vi "FipsAdjacent.vi"() -> (11 "Fips":i32[](array[numeric]))   [LabVIEW 2017] (continued)
County, MN\"\t27105\n\"Lyon County, IA\"\t19119\t\"Rock County, MN\"\t27133\n\"Lyon County, IA\"\t19119\t\"Lincoln County, SD\"\t46083\n\"Lyon County, IA\"\t19119\t\"Minnehaha County, SD\"\t46099\n\"Madison County, IA\"\t19121\t\"Adair County, IA\"\t19001\n\"Madison County, IA\"\t19121\t\"Clarke County, IA\"\t19039\n\"Madison County, IA\"\t19121\t\"Dallas County, IA\"\t19049\n\"Madison County, IA\"\t19121\t\"Guthrie County, IA\"\t19077\n\"Madison County, IA\"\t19121\t\"Madison County, IA\"\t19121\n\"Madison County, IA\"\t19121\t\"Polk County, IA\"\t19153\n\"Madison County, IA\"\t19121\t\"Union County, IA\"\t19175\n\"Madison County, IA\"\t19121\t\"Warren County, IA\"\t19181\n\"Mahaska County, IA\"\t19123\t\"Jasper County, IA\"\t19099\n\"Mahaska County, IA\"\t19123\t\"Keokuk County, IA\"\t19107\n\"Mahaska County, IA\"\t19123\t\"Mahaska County, IA\"\t19123\n\"Mahaska County, IA\"\t19123\t\"Marion County, IA\"\t19125\n\"Mahaska County, IA\"\t19123\t\"Monroe County, IA\"\t19135\n\"Mahaska County, IA\"\t19123\t\"Poweshiek County, IA\"\t19157\n\"Mahaska County, IA\"\t19123\t\"Wapello County, IA\"\t19179\n\"Marion County, IA\"\t19125\t\"Jasper County, IA\"\t19099\n\"Marion County, IA\"\t19125\t\"Lucas County, IA\"\t19117\n\"Marion County, IA\"\t19125\t\"Mahaska County, IA\"\t19123\n\"Marion County, IA\"\t19125\t\"Marion County, IA\"\t19125\n\"Marion County, IA\"\t19125\t\"Monroe County, IA\"\t19135\n\"Marion County, IA\"\t19125\t\"Polk County, IA\"\t19153\n\"Marion County, IA\"\t19125\t\"Warren County, IA\"\t19181\n\"Marshall County, IA\"\t19127\t\"Grundy County, IA\"\t19075\n\"Marshall County, IA\"\t19127\t\"Hardin County, IA\"\t19083\n\"Marshall County, IA\"\t19127\t\"Jasper County, IA\"\t19099\n\"Marshall County, IA\"\t19127\t\"Marshall County, IA\"\t19127\n\"Marshall County, IA\"\t19127\t\"Poweshiek County, IA\"\t19157\n\"Marshall County, IA\"\t19127\t\"Story County, IA\"\t19169\n\"Marshall County, IA\"\t19127\t\"Tama County, IA\"\t19171\n\"Mills County, IA\"\t19129\t\"Fremont County, IA\"\t19071\n\"Mills County, IA\"\t19129\t\"Mills County, IA\"\t19129\n\"Mills County, IA\"\t19129\t\"Montgomery County, IA\"\t19137\n\"Mills County, IA\"\t19129\t\"Page County, IA\"\t19145\n\"Mills County, IA\"\t19129\t\"Pottawattamie County, IA\"\t19155\n\"Mills County, IA\"\t19129\t\"Cass County, NE\"\t31025\n\"Mills County, IA\"\t19129\t\"Sarpy County, NE\"\t31153\n\"Mitchell County, IA\"\t19131\t\"Cerro Gordo County, IA\"\t19033\n\"Mitchell County, IA\"\t19131\t\"Chickasaw County, IA\"\t19037\n\"Mitchell County, IA\"\t19131\t\"Floyd County, IA\"\t19067\n\"Mitchell County, IA\"\t19131\t\"Howard County, IA\"\t19089\n\"Mitchell County, IA\"\t19131\t\"Mitchell County, IA\"\t19131\n\"Mitchell County, IA\"\t19131\t\"Worth County, IA\"\t19195\n\"Mitchell County, IA\"\t19131\t\"Mower County, MN\"\t27099\n\"Monona County, IA\"\t19133\t\"Crawford County, IA\"\t19047\n\"Monona County, IA\"\t19133\t\"Harrison County, IA\"\t19085\n\"Monona County, IA\"\t19133\t\"Ida County, IA\"\t19093\n\"Monona County, IA\"\t19133\t\"Monona County, IA\"\t19133\n\"Monona County, IA\"\t19133\t\"Woodbury County, IA\"\t19193\n\"Monona County, IA\"\t19133\t\"Burt County, NE\"\t31021\n\"Monona County, IA\"\t19133\t\"Thurston County, NE\"\t31173\n\"Monroe County, IA\"\t19135\t\"Appanoose County, IA\"\t19007\n\"Monroe County, IA\"\t19135\t\"Davis County, IA\"\t19051\n\"Monroe County, IA\"\t19135\t\"Lucas County, IA\"\t19117\n\"Monroe County, IA\"\t19135\t\"Mahaska County, IA\"\t19123\n\"Monroe County, IA\"\t19135\t\"Marion County, IA\"\t19125\n\"Monroe County, IA\"\t19135\t\"Monroe County, IA\"\t19135\n\"Monroe County, IA\"\t19135\t\"Wapello County, IA\"\t19179\n\"Monroe County, IA\"\t19135\t\"Wayne County, IA\"\t19185\n\"Montgomery County, IA\"\t19137\t\"Adams County, IA\"\t19003\n\"Montgomery County, IA\"\t19137\t\"Cass County, IA\"\t19029\n\"Montgomery County, IA\"\t19137\t\"Fremont County, IA\"\t19071\n\"Montgomery County, IA\"\t19137\t\"Mills County, IA\"\t19129\n\"Montgomery County, IA\"\t19137\t\"Montgomery County, IA\"\t19137\n\"Montgomery County, IA\"\t19137\t\"Page County, IA\"\t19145\n\"Montgomery County, IA\"\t19137\t\"Pottawattamie County, IA\"\t19155\n\"Montgomery County, IA\"\t19137\t\"Taylor County, IA\"\t19173\n\"Muscatine County, IA\"\t19139\t\"Rock Island County, IL\"\t17161\n\"Muscatine County, IA\"\t19139\t\"Cedar County, IA\"\t19031\n\"Muscatine County, IA\"\t19139\t\"Johnson County, IA\"\t19103\n\"Muscatine County, IA\"\t19139\t\"Louisa County, IA\"\t19115\n\"Muscatine County, IA\"\t19139\t\"Muscatine County, IA\"\t19139\n\"Muscatine County, IA\"\t19139\t\"Scott County, IA\"\t19163\n\"O'Brien County, IA\"\t19141\t\"Buena Vista County, IA\"\t19021\n\"O'Brien County, IA\"\t19141\t\"Cherokee County, IA\"\t19035\n\"O'Brien County, IA\"\t19141\t\"Clay County, IA\"\t19041\n\"O'Brien County, IA\"\t19141\t\"Dickinson County, IA\"\t19059\n\"O'Brien County, IA\"\t19141\t\"Lyon County, IA\"\t19119\n\"O'Brien County, IA\"\t19141\t\"O'Brien County, IA\"\t19141\n\"O'Brien County, IA\"\t19141\t\"Osceola County, IA\"\t19143\n\"O'Brien County, IA\"\t19141\t\"Plymouth County, IA\"\t19149\n\"O'Brien County, IA\"\t19141\t\"Sioux County, IA\"\t19167\n\"Osceola County, IA\"\t19143\t\"Clay County, IA\"\t19041\n\"Osceola County, IA\"\t19143\t\"Dickinson County, IA\"\t19059\n\"Osceola County, IA\"\t19143\t\"Lyon County, IA\"\t19119\n\"Osceola County, IA\"\t19143\t\"O'Brien County, IA\"\t19141\n\"Osceola County, IA\"\t19143\t\"Osceola County, IA\"\t19143\n\"Osceola County, IA\"\t19143\t\"Sioux County, IA\"\t19167\n\"Osceola County, IA\"\t19143\t\"Jackson County, MN\"\t27063\n\"Osceola County, IA\"\t19143\t\"Nobles County, MN\"\t27105\n\"Page County, IA\"\t19145\t\"Adams County, IA\"\t19003\n\"Page County, IA\"\t19145\t\"Fremont County, IA\"\t19071\n\"Page County, IA\"\t19145\t\"Mills County, IA\"\t19129\n\"Page County, IA\"\t19145\t\"Montgomery County, IA\"\t19137\n\"Page County, IA\"\t19145\t\"Page County, IA\"\t19145\n\"Page County, IA\"\t19145\t\"Taylor County, IA\"\t19173\n\"Page County, IA\"\t19145\t\"Atchison County, MO\"\t29005\n\"Page County, IA\"\t19145\t\"Nodaway County, MO\"\t29147\n\"Palo Alto County, IA\"\t19147\t\"Buena Vista County, IA\"\t19021\n\"Palo Alto County, IA\"\t19147\t\"Clay County, IA\"\t19041\n\"Palo Alto County, IA\"\t19147\t\"Dickinson County, IA\"\t19059\n\"Palo Alto County, IA\"\t19147\t\"Emmet County, IA\"\t19063\n\"Palo Alto County, IA\"\t19147\t\"Humboldt County, IA\"\t19091\n\"Palo Alto County, IA\"\t19147\t\"Kossuth County, IA\"\t19109\n\"Palo Alto County, IA\"\t19147\t\"Palo Alto County, IA\"\t19147\n\"Palo Alto County, IA\"\t19147\t\"Pocahontas County, IA\"\t19151\n\"Plymouth County, IA\"\t19149\t\"Cherokee County, IA\"\t19035\n\"Plymouth County, IA\"\t19149\t\"O'Brien County, IA\"\t19141\n\"Plymouth County, IA\"\t19149\t\"Plymouth County, IA\"\t19149\n\"Plymouth County, IA\"\t19149\t\"Sioux County, IA\"\t19167\n\"Plymouth County, IA\"\t19149\t\"Woodbury County, IA\"\t19193\n\"Plymouth County, IA\"\t19149\t\"Union County, SD\"\t46127\n\"Pocahontas County, IA\"\t19151\t\"Buena Vista County, IA\"\t19021\n\"Pocahontas County, IA\"\t19151\t\"Calhoun County, IA\"\t19025\n\"Pocahontas County, IA\"\t19151\t\"Clay County, IA\"\t19041\n\"Pocahontas County, IA\"\t19151\t\"Humboldt County, IA\"\t19091\n\"Pocahontas County, IA\"\t19151\t\"Kossuth County, IA\"\t19109\n\"Pocahontas County, IA\"\t19151\t\"Palo Alto County, IA\"\t19147\n\"Pocahontas County, IA\"\t19151\t\"Pocahontas County, IA\"\t19151\n\"Pocahontas County, IA\"\t19151\t\"Sac County, IA\"\t19161\n\"Pocahontas County, IA\"\t19151\t\"Webster County, IA\"\t19187\n\"Polk County, IA\"\t19153\t\"Boone County, IA\"\t19015\n\"Polk County, IA\"\t19153\t\"Dallas County, IA\"\t19049\n\"Polk County, IA\"\t19153\t\"Jasper County, IA\"\t19099\n\"Polk County, IA\"\t19153\t\"Madison County, IA\"\t19121\n\"Polk County, IA\"\t19153\t\"Marion County, IA\"\t19125\n\"Polk County, IA\"\t19153\t\"Polk County, IA\"\t19153\n\"Polk County, IA\"\t19153\t\"Story County, IA\"\t19169\n\"Polk County, IA\"\t19153\t\"Warren County, IA\"\t19181\n\"Pottawattamie County, IA\"\t19155\t\"Cass County, IA\"\t19029\n\"Pottawattamie County, IA\"\t19155\t\"Harrison County, IA\"\t19085\n\"Pottawattamie County, IA\"\t19155\t\"Mills County, IA\"\t19129\n\"Pottawattamie County, IA\"\t19155\t\"Montgomery County, IA\"\t19137\n\"Pottawattamie County, IA\"\t19155\t\"Pottawattamie County, IA\"\t19155\n\"Pottawattamie County, IA\"\t19155\t\"Shelby County, IA\"\t19165\n\"Pottawattamie County, IA\"\t19155\t\"Douglas County, NE\"\t31055\n\"Pottawattamie County, IA\"\t19155\t\"Sarpy County, NE\"\t31153\n\"Pottawattamie County, IA\"\t19155\t\"Washington County, NE\"\t31177\n\"Poweshiek County, IA\"\t19157\t\"Benton County, IA\"\t19011\n\"Poweshiek County, IA\"\t19157\t\"Iowa County, IA\"\t19095\n\"Poweshiek County, IA\"\t19157\t\"Jasper County, IA\"\t19099\n\"Poweshiek County, IA\"\t19157\t\"Keokuk County, IA\"\t19107\n\"Poweshiek County, IA\"\t19157\t\"Mahaska County, IA\"\t19123\n\"Poweshiek County, IA\"\t19157\t\"Marshall County, IA\"\t19127\n\"Poweshiek County, IA\"\t19157\t\"Poweshiek County, IA\"\t19157\n\"Poweshiek County, IA\"\t19157\t\"Tama County, IA\"\t19171\n\"Ringgold County, IA\"\t19159\t\"Adams County, IA\"\t19003\n\"Ringgold County, IA\"\t19159\t\"Clarke County, IA\"\t19039\n\"Ringgold County, IA\"\t19159\t\"Decatur County, IA\"\t19053\n\"Ringgold County, IA\"\t19159\t\"Ringgold County, IA\"\t19159\n\"Ringgold County, IA\"\t19159\t\"Taylor County, IA\"\t19173\n\"Ringgold County, IA\"\t19159\t\"Union County, IA\"\t19175\n\"Ringgold County, IA\"\t19159\t\"Harrison County, MO\"\t29081\n\"Ringgold County, IA\"\t19159\t\"Worth County, MO\"\t29227\n\"Sac County, IA\"\t19161\t\"Buena Vista County, IA\"\t19021\n\"Sac County, IA\"\t19161\t\"Calhoun County, IA\"\t19025\n\"Sac County, IA\"\t19161\t\"Carroll County, IA\"\t19027\n\"Sac County, IA\"\t19161\t\"Cherokee County, IA\"\t19035\n\"Sac County, IA\"\t19161\t\"Crawford County, IA\"\t19047\n\"Sac County, IA\"\t19161\t\"Ida County, IA\"\t19093\n\"Sac County, IA\"\t19161\t\"Pocahontas County, IA\"\t19151\n\"Sac County, IA\"\t19161\t\"Sac County, IA\"\t19161\n\"Scott County, IA\"\t19163\t\"Rock Island County, IL\"\t17161\n\"Scott County, IA\"\t19163\t\"Cedar County, IA\"\t19031\n\"Scott County, IA\"\t19163\t\"Clinton County, IA\"\t19045\n\"Scott County, IA\"\t19163\t\"Muscatine County, IA\"\t19139\n\"Scott County, IA\"\t19163\t\"Scott County, IA\"\t19163\n\"Shelby County, IA\"\t19165\t\"Audubon County, IA\"\t19009\n\"Shelby County, IA\"\t19165\t\"Carroll County, IA\"\t19027\n\"Shelby County, IA\"\t19165\t\"Cass County, IA\"\t19029\n\"Shelby County, IA\"\t19165\t\"Crawford County, IA\"\t19047\n\"Shelby County, IA\"\t19165\t\"Harrison County, IA\"\t19085\n\"Shelby County, IA\"\t19165\t\"Pottawattamie County, IA\"\t19155\n\"Shelby County, IA\"\t19165\t\"Shelby County, IA\"\t19165\n\"Sioux County, IA\"\t19167\t\"Cherokee County, IA\"\t19035\n\"Sioux County, IA\"\t19167\t\"Lyon County, IA\"\t19119\n\"Sioux County, IA\"\t19167\t\"O'Brien County, IA\"\t19141\n\"Sioux County, IA\"\t19167\t\"Osceola County, IA\"\t19143\n\"Sioux County, IA\"\t19167\t\"Plymouth County, IA\"\t19149\n\"Sioux County, IA\"\t19167\t\"Sioux County, IA\"\t19167\n\"Sioux County, IA\"\t19167\t\"Lincoln County, SD\"\t46083\n\"Sioux County, IA\"\t19167\t\"Union County, SD\"\t46127\n\"Story County, IA\"\t19169\t\"Boone County, IA\"\t19015\n\"Story County, IA\"\t19169\t\"Hamilton County, IA\"\t19079\n\"Story County, IA\"\t19169\t\"Hardin County, IA\"\t19083\n\"Story County, IA\"\t19169\t\"Jasper County, IA\"\t19099\n\"Story County, IA\"\t19169\t\"Marshall County, IA\"\t19127\n\"Story County, IA\"\t19169\t\"Polk County, IA\"\t19153\n\"Story County, IA\"\t19169\t\"Story County, IA\"\t19169\n\"Tama County, IA\"\t19171\t\"Benton County, IA\"\t19011\n\"Tama County, IA\"\t19171\t\"Black Hawk County, IA\"\t19013\n\"Tama County, IA\"\t19171\t\"Grundy County, IA\"\t19075\n\"Tama County, IA\"\t19171\t\"Iowa County, IA\"\t19095\n\"Tama County, IA\"\t19171\t\"Jasper County, IA\"\t19099\n\"Tama County, IA\"\t19171\t\"Marshall County, IA\"\t19127\n\"Tama County, IA\"\t19171\t\"Poweshiek County, IA\"\t19157\n\"Tama County, IA\"\t19171\t\"Tama County, IA\"\t19171\n\"Taylor County, IA\"\t19173\t\"Adams County, IA\"\t19003\n\"Taylor County, IA\"\t19173\t\"Montgomery County, IA\"\t19137\n\"Taylor County, IA\"\t19173\t\"Page County, IA\"\t19145\n\"Taylor County, IA\"\t19173\t\"Ringgold County, IA\"\t19159\n\"Taylor County, IA\"\t19173\t\"Taylor County, IA\"\t19173\n\"Taylor County, IA\"\t19173\t\"Union County, IA\"\t19175\n\"Taylor County, IA\"\t19173\t\"Nodaway County, MO\"\t29147\n\"Taylor County, IA\"\t19173\t\"Worth County, MO\"\t29227\n\"Union County, IA\"\t19175\t\"Adair County, IA\"\t19001\n\"Union County, IA\"\t19175\t\"Adams County, IA\"\t19003\n\"Union County, IA\"\t19175\t\"Clarke County, IA\"\t19039\n\"Union County, IA\"\t19175\t\"Decatur County, IA\"\t19053\n\"Union County, IA\"\t19175\t\"Madison County, IA\"\t19121\n\"Union County, IA\"\t19175\t\"Ringgold County, IA\"\t19159\n\"Union County, IA\"\t19175\t\"Taylor County, IA\"\t19173\n\"Union County, IA\"\t19175\t\"Union County, IA\"\t19175\n\"Van Buren County, IA\"\t19177\t\"Davis County, IA\"\t19051\n\"Van Buren County, IA\"\t19177\t\"Henry County, IA\"\t19087\n\"Van Buren County, IA\"\t19177\t\"Jefferson County, IA\"\t19101\n\"Van Buren County, IA\"\t19177\t\"Lee County, IA\"\t19111\n\"Van Buren County, IA\"\t19177\t\"Van Buren County, IA\"\t19177\n\"Van Buren County, IA\"\t19177\t\"Wapello County, IA\"\t19179\n\"Van Buren County, IA\"\t19177\t\"Clark County, MO\"\t29045\n\"Van Buren County, IA\"\t19177\t\"Scotland County, MO\"\t29199\n\"Wapello County, IA\"\t19179\t\"Appanoose County, IA\"\t19007\n\"Wapello County, IA\"\t19179\t\"Davis County, IA\"\t19051\n\"Wapello County, IA\"\t19179\t\"Jefferson County, IA\"\t19101\n\"Wapello County, IA\"\t19179\t\"Keokuk County, IA\"\t19107\n\"Wapello County, IA\"\t19179\t\"Mahaska County, IA\"\t19123\n\"Wapello County, IA\"\t19179\t\"Monroe County, IA\"\t19135\n\"Wapello County, IA\"\t19179\t\"Van Buren County, IA\"\t19177\n\"Wapello County, IA\"\t19179\t\"Wapello County, IA\"\t19179\n\"Warren County, IA\"\t19181\t\"Clarke County, IA\"\t19039\n\"Warren County, IA\"\t19181\t\"Dallas County, IA\"\t19049\n\"Warren County, IA\"\t19181\t\"Lucas County, IA\"\t19117\n\"Warren County, IA\"\t19181\t\"Madison County, IA\"\t19121\n\"Warren County, IA\"\t19181\t\"Marion County, IA\"\t19125\n\"Warren County, IA\"\t19181\t\"Polk County, IA\"\t19153\n\"Warren County, IA\"\t19181\t\"Warren County, IA\"\t19181\n\"Washington County, IA\"\t19183\t\"Henry County, IA\"\t19087\n\"Washington County, IA\"\t19183\t\"Iowa County, IA\"\t19095\n\"Washington County, IA\"\t19183\t\"Jefferson County, IA\"\t19101\n\"Washington County, IA\"\t19183\t\"Johnson County, IA\"\t19103\n\"Washington County, IA\"\t19183\t\"Keokuk County, IA\"\t19107\n\"Washington County, IA\"\t19183\t\"Louisa County, IA\"\t19115\n\"Washington County, IA\"\t19183\t\"Washington County, IA\"\t19183\n\"Wayne County, IA\"\t19185\t\"Appanoose County, IA\"\t19007\n\"Wayne County, IA\"\t19185\t\"Clarke County, IA\"\t19039\n\"Wayne County, IA\"\t19185\t\"Decatur County, IA\"\t19053\n\"Wayne County, IA\"\t19185\t\"Lucas County, IA\"\t19117\n\"Wayne County, IA\"\t19185\t\"Monroe County, IA\"\t19135\n\"Wayne County, IA\"\t19185\t\"Wayne County, IA\"\t19185\n\"Wayne County, IA\"\t19185\t\"Mercer County, MO\"\t29129\n\"Wayne County, IA\"\t19185\t\"Putnam County, MO\"\t29171\n\"Webster County, IA\"\t19187\t\"Boone County, IA\"\t19015\n\"Webster County, IA\"\t19187\t\"Calhoun County, IA\"\t19025\n\"Webster County, IA\"\t19187\t\"Greene County, IA\"\t19073\n\"Webster County, IA\"\t19187\t\"Hamilton County, IA\"\t19079\n\"Webster County, IA\"\t19187\t\"Humboldt County, IA\"\t19091\n\"Webster County, IA\"\t19187\t\"Pocahontas County, IA\"\t19151\n\"Webster County, IA\"\t19187\t\"Webster County, IA\"\t19187\n\"Webster County, IA\"\t19187\t\"Wright County, IA\"\t19197\n\"Winnebago County, IA\"\t19189\t\"Cerro Gordo County, IA\"\t19033\n\"Winnebago County, IA\"\t19189\t\"Hancock County, IA\"\t19081\n\"Winnebago County, IA\"\t19189\t\"Kossuth County, IA\"\t19109\n\"Winnebago County, IA\"\t19189\t\"Winnebago County, IA\"\t19189\n\"Winnebago County, IA\"\t19189\t\"Worth County, IA\"\t19195\n\"Winnebago County, IA\"\t19189\t\"Faribault County, MN\"\t27043\n\"Winnebago County, IA\"\t19189\t\"Freeborn County, MN\"\t27047\n\"Winneshiek County, IA\"\t19191\t\"Allamakee County, IA\"\t19005\n\"Winneshiek County, IA\"\t19191\t\"Chickasaw County, IA\"\t19037\n\"Winneshiek County, IA\"\t19191\t\"Clayton County, IA\"\t19043\n\"Winneshiek County, IA\"\t19191\t\"Fayette County, IA\"\t19065\n\"Winneshiek County, IA\"\t19191\t\"Howard County, IA\"\t19089\n\"Winneshiek County, IA\"\t19191\t\"Winneshiek County, IA\"\t19191\n\"Winneshiek County, IA\"\t19191\t\"Fillmore County, MN\"\t27045\n\"Winneshiek County, IA\"\t19191\t\"Houston County, MN\"\t27055\n\"Woodbury County, IA\"\t19193\t\"Cherokee County, IA\"\t19035\n\"Woodbury County, IA\"\t19193\t\"Crawford County, IA\"\t19047\n\"Woodbury County, IA\"\t19193\t\"Ida County, IA\"\t19093\n\"Woodbury County, IA\"\t19193\t\"Monona County, IA\"\t19133\n\"Woodbury County, IA\"\t19193\t\"Plymouth County, IA\"\t19149\n\"Woodbury County, IA\"\t19193\t\"Woodbury County, IA\"\t19193\n\"Woodbury County, IA\"\t19193\t\"Dakota County, NE\"\t31043\n\"Woodbury County, IA\"\t19193\t\"Thurston County, NE\"\t31173\n\"Woodbury County, IA\"\t19193\t\"Union County, SD\"\t46127\n\"Worth County, IA\"\t19195\t\"Cerro Gordo County, IA\"\t19033\n\"Worth County, IA\"\t19195\t\"Hancock County, IA\"\t19081\n\"Worth County, IA\"\t19195\t\"Mitchell County, IA\"\t19131\n\"Worth County, IA\"\t19195\t\"Winnebago County, IA\"\t19189\n\"Worth County, IA\"\t19195\t\"Worth County, IA\"\t19195\n\"Worth County, IA\"\t19195\t\"Freeborn County, MN\"\t27047\n\"Worth County, IA\"\t19195\t\"Mower County, MN\"\t27099\n\"Wright County, IA\"\t19197\t\"Cerro Gordo County, IA\"\t19033\n\"Wright County, IA\"\t19197\t\"Franklin County, IA\"\t19069\n\"Wright County, IA\"\t19197\t\"Hamilton County, IA\"\t19079\n\"Wright County, IA\"\t19197\t\"Hancock County, IA\"\t19081\n\"Wright County, IA\"\t19197\t\"Hardin County, IA\"\t19083\n\"Wright County, IA\"\t19197\t\"Humboldt County, IA\"\t19091\n\"Wright County, IA\"\t19197\t\"Kossuth County, IA\"\t19109\n\"Wright County, IA\"\t19197\t\"Webster County, IA\"\t19187\n\"Wright County, IA\"\t19197\t\"Wright County, IA\"\t19197\n\"Allen County, KS\"\t20001\t\"Allen County, KS\"\t20001\n\"Allen County, KS\"\t20001\t\"Anderson County, KS\"\t20003\n\"Allen County, KS\"\t20001\t\"Bourbon County, KS\"\t20011\n\"Allen County, KS\"\t20001\t\"Coffey County, KS\"\t20031\n\"Allen County, KS\"\t20001\t\"Linn County, KS\"\t20107\n\"Allen County, KS\"\t20001\t\"Neosho County, KS\"\t20133\n\"Allen County, KS\"\t20001\t\"Wilson County, KS\"\t20205\n\"Allen County, KS\"\t20001\t\"Woodson County, KS\"\t20207\n\"Anderson County, KS\"\t20003\t\"Allen County, KS\"\t20001\n\"Anderson County, KS\"\t20003\t\"Anderson County, KS\"\t20003\n\"Anderson County, KS\"\t20003\t\"Bourbon County, KS\"\t20011\n\"Anderson County, KS\"\t20003\t\"Coffey County, KS\"\t20031\n\"Anderson County, KS\"\t20003\t\"Franklin County, KS\"\t20059\n\"Anderson County, KS\"\t20003\t\"Linn County, KS\"\t20107\n\"Anderson County, KS\"\t20003\t\"Miami County, KS\"\t20121\n\"Anderson County, KS\"\t20003\t\"Woodson County, KS\"\t20207\n\"Atchison County, KS\"\t20005\t\"Atchison County, KS\"\t20005\n\"Atchison County, KS\"\t20005\t\"Brown County, KS\"\t20013\n\"Atchison County, KS\"\t20005\t\"Doniphan County, KS\"\t20043\n\"Atchison County, KS\"\t20005\t\"Jackson County, KS\"\t20085\n\"Atchison County, KS\"\t20005\t\"Jefferson County, KS\"\t20087\n\"Atchison County, KS\"\t20005\t\"Leavenworth County, KS\"\t20103\n\"Atchison County, KS\"\t20005\t\"Buchanan County, MO\"\t29021\n\"Atchison County, KS\"\t20005\t\"Platte County, MO\"\t29165\n\"Barber County, KS\"\t20007\t\"Barber County, KS\"\t20007\n\"Barber County, KS\"\t20007\t\"Comanche County, KS\"\t20033\n\"Barber County, KS\"\t20007\t\"Harper County, KS\"\t20077\n\"Barber County, KS\"\t20007\t\"Kingman County, KS\"\t20095\n\"Barber County, KS\"\t20007\t\"Kiowa County, KS\"\t20097\n\"Barber County, KS\"\t20007\t\"Pratt County, KS\"\t20151\n\"Barber County, KS\"\t20007\t\"Alfalfa County, OK\"\t40003\n\"Barber County, KS\"\t20007\t\"Woods County, OK\"\t40151\n\"Barton County, KS\"\t20009\t\"Barton County, KS\"\t20009\n\"Barton County, KS\"\t20009\t\"Ellsworth County, KS\"\t20053\n\"Barton County, KS\"\t20009\t\"Pawnee County, KS\"\t20145\n\"Barton County, KS\"\t20009\t\"Rice County, KS\"\t20159\n\"Barton County, KS\"\t20009\t\"Rush County, KS\"\t20165\n\"Barton County, KS\"\t20009\t\"Russell County, KS\"\t20167\n\"Barton County, KS\"\t20009\t\"Stafford County, KS\"\t20185\n\"Bourbon County, KS\"\t20011\t\"Allen County, KS\"\t20001\n\"Bourbon County, KS\"\t20011\t\"Anderson County, KS\"\t20003\n\"Bourbon County, KS\"\t20011\t\"Bourbon County, KS\"\t20011\n\"Bourbon County, KS\"\t20011\t\"Crawford County, KS\"\t20037\n\"Bourbon County, KS\"\t20011\t\"Linn County, KS\"\t20107\n\"Bourbon County, KS\"\t20011\t\"Neosho County, KS\"\t20133\n\"Bourbon County, KS\"\t20011\t\"Vernon County, MO\"\t29217\n\"Brown County, KS\"\t20013\t\"Atchison County, KS\"\t20005\n\"Brown County, KS\"\t20013\t\"Brown County, KS\"\t20013\n\"Brown County, KS\"\t20013\t\"Doniphan County, KS\"\t20043\n\"Brown County, KS\"\t20013\t\"Jackson County, KS\"\t20085\n\"Brown County, KS\"\t20013\t\"Nemaha County, KS\"\t20131\n\"Brown County, KS\"\t20013\t\"Richardson County, NE\"\t31147\n\"Butler County, KS\"\t20015\t\"Butler County, KS\"\t20015\n\"Butler County, KS\"\t20015\t\"Chase County, KS\"\t20017\n\"Butler County, KS\"\t20015\t\"Cowley County, KS\"\t20035\n\"Butler County, KS\"\t20015\t\"Elk County, KS\"\t20049\n\"Butler County, KS\"\t20015\t\"Greenwood County, KS\"\t20073\n\"Butler County, KS\"\t20015\t\"Harvey County, KS\"\t20079\n\"Butler County, KS\"\t20015\t\"Marion County, KS\"\t20115\n\"Butler County, KS\"\t20015\t\"Sedgwick County, KS\"\t20173\n\"Butler County, KS\"\t20015\t\"Sumner County, KS\"\t20191\n\"Chase County, KS\"\t20017\t\"Butler County, KS\"\t20015\n\"Chase County, KS\"\t20017\t\"Chase County, KS\"\t20017\n\"Chase County, KS\"\t20017\t\"Greenwood County, KS\"\t20073\n\"Chase County, KS\"\t20017\t\"Lyon County, KS\"\t20111\n\"Chase County, KS\"\t20017\t\"Marion County, KS\"\t20115\n\"Chase County, KS\"\t20017\t\"Morris County, KS\"\t20127\n\"Chautauqua County, KS\"\t20019\t\"Chautauqua County, KS\"\t20019\n\"Chautauqua County, KS\"\t20019\t\"Cowley County, KS\"\t20035\n\"Chautauqua County, KS\"\t20019\t\"Elk County, KS\"\t20049\n\"Chautauqua County, KS\"\t20019\t\"Montgomery County, KS\"\t20125\n\"Chautauqua County, KS\"\t20019\t\"Osage County, OK\"\t40113\n\"Chautauqua County, KS\"\t20019\t\"Washington County, OK\"\t40147\n\"Cherokee County, KS\"\t20021\t\"Cherokee County, KS\"\t20021\n\"Cherokee County, KS\"\t20021\t\"Crawford County, KS\"\t20037\n\"Cherokee County, KS\"\t20021\t\"Labette County, KS\"\t20099\n\"Cherokee County, KS\"\t20021\t\"Jasper County, MO\"\t29097\n\"Cherokee County, KS\"\t20021\t\"Newton County, MO\"\t29145\n\"Cherokee County, KS\"\t20021\t\"Craig County, OK\"\t40035\n\"Cherokee County, KS\"\t20021\t\"Ottawa County, OK\"\t40115\n\"Cheyenne County, KS\"\t20023\t\"Kit Carson County, CO\"\t08063\n\"Cheyenne County, KS\"\t20023\t\"Yuma County, CO\"\t08125\n\"Cheyenne County, KS\"\t20023\t\"Cheyenne County, KS\"\t20023\n\"Cheyenne County, KS\"\t20023\t\"Rawlins County, KS\"\t20153\n\"Cheyenne County, KS\"\t20023\t\"Sherman County, KS\"\t20181\n\"Cheyenne County, KS\"\t20023\t\"Dundy County, NE\"\t31057\n\"Clark County, KS\"\t20025\t\"Clark County, KS\"\t20025\n\"Clark County, KS\"\t20025\t\"Comanche County, KS\"\t20033\n\"Clark County, KS\"\t20025\t\"Ford County, KS\"\t20057\n\"Clark County, KS\"\t20025\t\"Kiowa County, KS\"\t20097\n\"Clark County, KS\"\t20025\t\"Meade County, KS\"\t20119\n\"Clark County, KS\"\t20025\t\"Beaver County, OK\"\t40007\n\"Clark County, KS\"\t20025\t\"Harper County, OK\"\t40059\n\"Clay County, KS\"\t20027\t\"Clay County, KS\"\t20027\n\"Clay County, KS\"\t20027\t\"Cloud County, KS\"\t20029\n\"Clay County, KS\"\t20027\t\"Dickinson County, KS\"\t20041\n\"Clay County, KS\"\t20027\t\"Geary County, KS\"\t20061\n\"Clay County, KS\"\t20027\t\"Ottawa County, KS\"\t20143\n\"Clay County, KS\"\t20027\t\"Riley County, KS\"\t20161\n\"Clay County, KS\"\t20027\t\"Washington County, KS\"\t20201\n\"Cloud County, KS\"\t20029\t\"Clay County, KS\"\t20027\n\"Cloud County, KS\"\t20029\t\"Cloud County, KS\"\t20029\n\"Cloud County, KS\"\t20029\t\"Jewell County, KS\"\t20089\n\"Cloud County, KS\"\t20029\t\"Mitchell County, KS\"\t20123\n\"Cloud County, KS\"\t20029\t\"Ottawa County, KS\"\t20143\n\"Cloud County, KS\"\t20029\t\"Republic County, KS\"\t20157\n\"Cloud County, KS\"\t20029\t\"Washington County, KS\"\t20201\n\"Coffey County, KS\"\t20031\t\"Allen County, KS\"\t20001\n\"Coffey County, KS\"\t20031\t\"Anderson County, KS\"\t20003\n\"Coffey County, KS\"\t20031\t\"Coffey County, KS\"\t20031\n\"Coffey County, KS\"\t20031\t\"Franklin County, KS\"\t20059\n\"Coffey County, KS\"\t20031\t\"Greenwood County, KS\"\t20073\n\"Coffey County, KS\"\t20031\t\"Lyon County, KS\"\t20111\n\"Coffey County, KS\"\t20031\t\"Osage County, KS\"\t20139\n\"Coffey County, KS\"\t20031\t\"Woodson County, KS\"\t20207\n\"Comanche County, KS\"\t20033\t\"Barber County, KS\"\t20007\n\"Comanche County, KS\"\t20033\t\"Clark County, KS\"\t20025\n\"Comanche County, KS\"\t20033\t\"Comanche County, KS\"\t20033\n\"Comanche County, KS\"\t20033\t\"Kiowa County, KS\"\t20097\n\"Comanche County, KS\"\t20033\t\"Harper County, OK\"\t40059\n\"Comanche County, KS\"\t20033\t\"Woods County, OK\"\t40151\n\"Cowley County, KS\"\t20035\t\"Butler County, KS\"\t20015\n\"Cowley County, KS\"\t20035\t\"Chautauqua County, KS\"\t20019\n\"Cowley County, KS\"\t20035\t\"Cowley County, KS\"\t20035\n\"Cowley County, KS\"\t20035\t\"Elk County, KS\"\t20049\n\"Cowley County, KS\"\t20035\t\"Sedgwick County, KS\"\t20173\n\"Cowley County, KS\"\t20035\t\"Sumner County, KS\"\t20191\n\"Cowley County, KS\"\t20035\t\"Kay County, OK\"\t40071\n\"Cowley County, KS\"\t20035\t\"Osage County, OK\"\t40113\n\"Crawford County, KS\"\t20037\t\"Bourbon County, KS\"\t20011\n\"Crawford County, KS\"\t20037\t\"Cherokee County, KS\"\t20021\n\"Crawford County, KS\"\t20037\t\"Crawford County, KS\"\t20037\n\"Crawford County, KS\"\t20037\t\"Labette County, KS\"\t20099\n\"Crawford County, KS\"\t20037\t\"Neosho County, KS\"\t20133\n\"Crawford County, KS\"\t20037\t\"Barton County, MO\"\t29011\n\"Crawford County, KS\"\t20037\t\"Jasper County, MO\"\t29097\n\"Crawford County, KS\"\t20037\t\"Vernon County, MO\"\t29217\n\"Decatur County, KS\"\t20039\t\"Decatur County, KS\"\t20039\n\"Decatur County, KS\"\t20039\t\"Norton County, KS\"\t20137\n\"Decatur County, KS\"\t20039\t\"Rawlins County, KS\"\t20153\n\"Decatur County, KS\"\t20039\t\"Sheridan County, KS\"\t20179\n\"Decatur County, KS\"\t20039\t\"Thomas County, KS\"\t20193\n\"Decatur County, KS\"\t20039\t\"Furnas County, NE\"\t31065\n\"Decatur County, KS\"\t20039\t\"Red Willow County, NE\"\t31145\n\"Dickinson County, KS\"\t20041\t\"Clay County, KS\"\t20027\n\"Dickinson County, KS\"\t20041\t\"Dickinson County, KS\"\t20041\n\"Dickinson County, KS\"\t20041\t\"Geary County, KS\"\t20061\n\"Dickinson County, KS\"\t20041\t\"McPherson County, KS\"\t20113\n\"Dickinson County, KS\"\t20041\t\"Marion County, KS\"\t20115\n\"Dickinson County, KS\"\t20041\t\"Morris County, KS\"\t20127\n\"Dickinson County, KS\"\t20041\t\"Ottawa County, KS\"\t20143\n\"Dickinson County, KS\"\t20041\t\"Saline County, KS\"\t20169\n\"Doniphan County, KS\"\t20043\t\"Atchison County, KS\"\t20005\n\"Doniphan County, KS\"\t20043\t\"Brown County, KS\"\t20013\n\"Doniphan County, KS\"\t20043\t\"Doniphan County, KS\"\t20043\n\"Doniphan County, KS\"\t20043\t\"Andrew County, MO\"\t29003\n\"Doniphan County, KS\"\t20043\t\"Buchanan County, MO\"\t29021\n\"Doniphan County, KS\"\t20043\t\"Holt County, MO\"\t29087\n\"Doniphan County, KS\"\t20043\t\"Richardson County, NE\"\t31147\n\"Douglas County, KS\"\t20045\t\"Douglas County, KS\"\t20045\n\"Douglas County, KS\"\t20045\t\"Franklin County, KS\"\t20059\n\"Douglas County, KS\"\t20045\t\"Jefferson County, KS\"\t20087\n\"Douglas County, KS\"\t20045\t\"Johnson County, KS\"\t20091\n\"Douglas County, KS\"\t20045\t\"Leavenworth County, KS\"\t20103\n\"Douglas County, KS\"\t20045\t\"Miami County, KS\"\t20121\n\"Douglas County, KS\"\t20045\t\"Osage County, KS\"\t20139\n\"Douglas County, KS\"\t20045\t\"Shawnee County, KS\"\t20177\n\"Edwards County, KS\"\t20047\t\"Edwards County, KS\"\t20047\n\"Edwards County, KS\"\t20047\t\"Ford County, KS\"\t20057\n\"Edwards County, KS\"\t20047\t\"Hodgeman County, KS\"\t20083\n\"Edwards County, KS\"\t20047\t\"Kiowa County, KS\"\t20097\n\"Edwards County, KS\"\t20047\t\"Pawnee County, KS\"\t20145\n\"Edwards County, KS\"\t20047\t\"Pratt County, KS\"\t20151\n\"Edwards County, KS\"\t20047\t\"Stafford County, KS\"\t20185\n\"Elk County, KS\"\t20049\t\"Butler County, KS\"\t20015\n\"Elk County, KS\"\t20049\t\"Chautauqua County, KS\"\t20019\n\"Elk County, KS\"\t20049\t\"Cowley County, KS\"\t20035\n\"Elk County, KS\"\t20049\t\"Elk County, KS\"\t20049\n\"Elk County, KS\"\t20049\t\"Greenwood County, KS\"\t20073\n\"Elk County, KS\"\t20049\t\"Montgomery County, KS\"\t20125\n\"Elk County, KS\"\t20049\t\"Wilson County, KS\"\t20205\n\"Ellis County, KS\"\t20051\t\"Ellis County, KS\"\t20051\n\"Ellis County, KS\"\t20051\t\"Ness County, KS\"\t20135\n\"Ellis County, KS\"\t20051\t\"Osborne County, KS\"\t20141\n\"Ellis County, KS\"\t20051\t\"Rooks County, KS\"\t20163\n\"Ellis County, KS\"\t20051\t\"Rush County, KS\"\t20165\n\"Ellis County, KS\"\t20051\t\"Russell County, KS\"\t20167\n\"Ellis County, KS\"\t20051\t\"Trego County, KS\"\t20195\n\"Ellsworth County, KS\"\t20053\t\"Barton County, KS\"\t20009\n\"Ellsworth County, KS\"\t20053\t\"Ellsworth County, KS\"\t20053\n\"Ellsworth County, KS\"\t20053\t\"Lincoln County, KS\"\t20105\n\"Ellsworth County, KS\"\t20053\t\"McPherson County, KS\"\t20113\n\"Ellsworth County, KS\"\t20053\t\"Rice County, KS\"\t20159\n\"Ellsworth County, KS\"\t20053\t\"Russell County, KS\"\t20167\n\"Ellsworth County, KS\"\t20053\t\"Saline County, KS\"\t20169\n\"Finney County, KS\"\t20055\t\"Finney County, KS\"\t20055\n\"Finney County, KS\"\t20055\t\"Grant County, KS\"\t20067\n\"Finney County, KS\"\t20055\t\"Gray County, KS\"\t20069\n\"Finney County, KS\"\t20055\t\"Haskell County, KS\"\t20081\n\"Finney County, KS\"\t20055\t\"Hodgeman County, KS\"\t20083\n\"Finney County, KS\"\t20055\t\"Kearny County, KS\"\t20093\n\"Finney County, KS\"\t20055\t\"Lane County, KS\"\t20101\n\"Finney County, KS\"\t20055\t\"Ness County, KS\"\t20135\n\"Finney County, KS\"\t20055\t\"Scott County, KS\"\t20171\n\"Ford County, KS\"\t20057\t\"Clark County, KS\"\t20025\n\"Ford County, KS\"\t20057\t\"Edwards County, KS\"\t20047\n\"Ford County, KS\"\t20057\t\"Ford County, KS\"\t20057\n\"Ford County, KS\"\t20057\t\"Gray County, KS\"\t20069\n\"Ford County, KS\"\t20057\t\"Hodgeman County, KS\"\t20083\n\"Ford County, KS\"\t20057\t\"Kiowa County, KS\"\t20097\n\"Ford County, KS\"\t20057\t\"Meade County, KS\"\t20119\n\"Franklin County, KS\"\t20059\t\"Anderson County, KS\"\t20003\n\"Franklin County, KS\"\t20059\t\"Coffey County, KS\"\t20031\n\"Franklin County, KS\"\t20059\t\"Douglas County, KS\"\t20045\n\"Franklin County, KS\"\t20059\t\"Franklin County, KS\"\t20059\n\"Franklin County, KS\"\t20059\t\"Johnson County, KS\"\t20091\n\"Franklin County, KS\"\t20059\t\"Linn County, KS\"\t20107\n\"Franklin County, KS\"\t20059\t\"Miami County, KS\"\t20121\n\"Franklin County, KS\"\t20059\t\"Osage County, KS\"\t20139\n\"Geary County, KS\"\t20061\t\"Clay County, KS\"\t20027\n\"Geary County, KS\"\t20061\t\"Dickinson County, KS\"\t20041\n\"Geary County, KS\"\t20061\t\"Geary County, KS\"\t20061\n\"Geary County, KS\"\t20061\t\"Morris County, KS\"\t20127\n\"Geary County, KS\"\t20061\t\"Riley County, KS\"\t20161\n\"Geary County, KS\"\t20061\t\"Wabaunsee County, KS\"\t20197\n\"Gove County, KS\"\t20063\t\"Gove County, KS\"\t20063\n\"Gove County, KS\"\t20063\t\"Graham County, KS\"\t20065\n\"Gove County, KS\"\t20063\t\"Lane County, KS\"\t20101\n\"Gove County, KS\"\t20063\t\"Logan County, KS\"\t20109\n\"Gove County, KS\"\t20063\t\"Ness County, KS\"\t20135\n\"Gove County, KS\"\t20063\t\"Scott County, KS\"\t20171\n\"Gove County, KS\"\t20063\t\"Sheridan County, KS\"\t20179\n\"Gove County, KS\"\t20063\t\"Thomas County, KS\"\t20193\n\"Gove County, KS\"\t20063\t\"Trego County, KS\"\t20195\n\"Graham County, KS\"\t20065\t\"Gove County, KS\"\t20063\n\"Graham County, KS\"\t20065\t\"Graham County, KS\"\t20065\n\"Graham County, KS\"\t20065\t\"Norton County, KS\"\t20137\n\"Graham County, KS\"\t20065\t\"Phillips County, KS\"\t20147\n\"Graham County, KS\"\t20065\t\"Rooks County, KS\"\t20163\n\"Graham County, KS\"\t20065\t\"Sheridan County, KS\"\t20179\n\"Graham County, KS\"\t20065\t\"Trego County, KS\"\t20195\n\"Grant County, KS\"\t20067\t\"Finney County, KS\"\t20055\n\"Grant County, KS\"\t20067\t\"Grant County, KS\"\t20067\n\"Grant County, KS\"\t20067\t\"Hamilton County, KS\"\t20075\n\"Grant County, KS\"\t20067\t\"Haskell County, KS\"\t20081\n\"Grant County, KS\"\t20067\t\"Kearny County, KS\"\t20093\n\"Grant County, KS\"\t20067\t\"Stanton County, KS\"\t20187\n\"Grant County, KS\"\t20067\t\"Stevens County, KS\"\t20189\n\"Gray County, KS\"\t20069\t\"Finney County, KS\"\t20055\n\"Gray County, KS\"\t20069\t\"Ford County, KS\"\t20057\n\"Gray County, KS\"\t20069\t\"Gray County, KS\"\t20069\n\"Gray County, KS\"\t20069\t\"Haskell County, KS\"\t20081\n\"Gray County, KS\"\t20069\t\"Hodgeman County, KS\"\t20083\n\"Gray County, KS\"\t20069\t\"Meade County, KS\"\t20119\n\"Greeley County, KS\"\t20071\t\"Cheyenne County, CO\"\t08017\n\"Greeley County, KS\"\t20071\t\"Kiowa County, CO\"\t08061\n\"Greeley County, KS\"\t20071\t\"Prowers County, CO\"\t08099\n\"Greeley County, KS\"\t20071\t\"Greeley County, KS\"\t20071\n\"Greeley County, KS\"\t20071\t\"Hamilton County, KS\"\t20075\n\"Greeley County, KS\"\t20071\t\"Wallace County, KS\"\t20199\n\"Greeley County, KS\"\t20071\t\"Wichita County, KS\"\t20203\n\"Greenwood County, KS\"\t20073\t\"Butler County, KS\"\t20015\n\"Greenwood County, KS\"\t20073\t\"Chase County, KS\"\t20017\n\"Greenwood County, KS\"\t20073\t\"Coffey County, KS\"\t20031\n\"Greenwood County, KS\"\t20073\t\"Elk County, KS\"\t20049\n\"Greenwood County, KS\"\t20073\t\"Greenwood County, KS\"\t20073\n\"Greenwood County, KS\"\t20073\t\"Lyon County, KS\"\t20111\n\"Greenwood County, KS\"\t20073\t\"Wilson County, KS\"\t20205\n\"Greenwood County, KS\"\t20073\t\"Woodson County, KS\"\t20207\n\"Hamilton County, KS\"\t20075\t\"Prowers County, CO\"\t08099\n\"Hamilton County, KS\"\t20075\t\"Grant County, KS\"\t20067\n\"Hamilton County, KS\"\t20075\t\"Greeley County, KS\"\t20071\n\"Hamilton County, KS\"\t20075\t\"Hamilton County, KS\"\t20075\n\"Hamilton County, KS\"\t20075\t\"Kearny County, KS\"\t20093\n\"Hamilton County, KS\"\t20075\t\"Stanton County, KS\"\t20187\n\"Hamilton County, KS\"\t20075\t\"Wichita County, KS\"\t20203\n\"Harper County, KS\"\t20077\t\"Barber County, KS\"\t20007\n\"Harper County, KS\"\t20077\t\"Harper County, KS\"\t20077\n\"Harper County, KS\"\t20077\t\"Kingman County, KS\"\t20095\n\"Harper County, KS\"\t20077\t\"Sumner County, KS\"\t20191\n\"Harper County, KS\"\t20077\t\"Alfalfa County, OK\"\t40003\n\"Harper County, KS\"\t20077\t\"Grant County, OK\"\t40053\n\"Harvey County, KS\"\t20079\t\"Butler County, KS\"\t20015\n\"Harvey County, KS\"\t20079\t\"Harvey County, KS\"\t20079\n\"Harvey County, KS\"\t20079\t\"McPherson County, KS\"\t20113\n\"Harvey County, KS\"\t20079\t\"Marion County, KS\"\t20115\n\"Harvey County, KS\"\t20079\t\"Reno County, KS\"\t20155\n\"Harvey County, KS\"\t20079\t\"Sedgwick County, KS\"\t20173\n\"Haskell County, KS\"\t20081\t\"Finney County, KS\"\t20055\n\"Haskell County, KS\"\t20081\t\"Grant County, KS\"\t20067\n\"Haskell County, KS\"\t20081\t\"Gray County, KS\"\t20069\n\"Haskell County, KS\"\t20081\t\"Haskell County, KS\"\t20081\n\"Haskell County, KS\"\t20081\t\"Kearny County, KS\"\t20093\n\"Haskell County, KS\"\t20081\t\"Meade County, KS\"\t20119\n\"Haskell County, KS\"\t20081\t\"Seward County, KS\"\t20175\n\"Haskell County, KS\"\t20081\t\"Stevens County, KS\"\t20189\n\"Hodgeman County, KS\"\t20083\t\"Edwards County, KS\"\t20047\n\"Hodgeman County, KS\"\t20083\t\"Finney County, KS\"\t20055\n\"Hodgeman County, KS\"\t20083\t\"Ford County, KS\"\t20057\n\"Hodgeman County, KS\"\t20083\t\"Gray County, KS\"\t20069\n\"Hodgeman County, KS\"\t20083\t\"Hodgeman County, KS\"\t20083\n\"Hodgeman County, KS\"\t20083\t\"Ness County, KS\"\t20135\n\"Hodgeman County, KS\"\t20083\t\"Pawnee County, KS\"\t20145\n\"Jackson County, KS\"\t20085\t\"Atchison County, KS\"\t20005\n\"Jackson County, KS\"\t20085\t\"Brown County, KS\"\t20013\n\"Jackson County, KS\"\t20085\t\"Jackson County, KS\"\t20085\n\"Jackson County, KS\"\t20085\t\"Jefferson County, KS\"\t20087\n\"Jackson County, KS\"\t20085\t\"Nemaha County, KS\"\t20131\n\"Jackson County, KS\"\t20085\t\"Pottawatomie County, KS\"\t20149\n\"Jackson County, KS\"\t20085\t\"Shawnee County, KS\"\t20177\n\"Jefferson County, KS\"\t20087\t\"Atchison County, KS\"\t20005\n\"Jefferson County, KS\"\t20087\t\"Douglas County, KS\"\t20045\n\"Jefferson County, KS\"\t20087\t\"Jackson County, KS\"\t20085\n\"Jefferson County, KS\"\t20087\t\"Jefferson County, KS\"\t20087\n\"Jefferson County, KS\"\t20087\t\"Leavenworth County, KS\"\t20103\n\"Jefferson County, KS\"\t20087\t\"Shawnee County, KS\"\t20177\n\"Jewell County, KS\"\t20089\t\"Cloud County, KS\"\t20029\n\"Jewell County, KS\"\t20089\t\"Jewell County, KS\"\t20089\n\"Jewell County, KS\"\t20089\t\"Mitchell County, KS\"\t20123\n\"Jewell County, KS\"\t20089\t\"Osborne County, KS\"\t20141\n\"Jewell County, KS\"\t20089\t\"Republic County, KS\"\t20157\n\"Jewell County, KS\"\t20089\t\"Smith County, KS\"\t20183\n\"Jewell County, KS\"\t20089\t\"Nuckolls County, NE\"\t31129\n\"Jewell County, KS\"\t20089\t\"Webster County, NE\"\t31181\n\"Johnson County, KS\"\t20091\t\"Douglas County, KS\"\t20045\n\"Johnson County, KS\"\t20091\t\"Franklin County, KS\"\t20059\n\"Johnson County, KS\"\t20091\t\"Johnson County, KS\"\t20091\n\"Johnson County, KS\"\t20091\t\"Leavenworth County, KS\"\t20103\n\"Johnson County, KS\"\t20091\t\"Miami County, KS\"\t20121\n\"Johnson County, KS\"\t20091\t\"Wyandotte County, KS\"\t20209\n\"Johnson County, KS\"\t20091\t\"Cass County, MO\"\t29037\n\"Johnson County, KS\"\t20091\t\"Jackson County, MO\"\t29095\n\"Kearny County, KS\"\t20093\t\"Finney County, KS\"\t20055\n\"Kearny County, KS\"\t20093\t\"Grant County, KS\"\t20067\n\"Kearny County, KS\"\t20093\t\"Hamilton County, KS\"\t20075\n\"Kearny County, KS\"\t20093\t\"Haskell County, KS\"\t20081\n\"Kearny County, KS\"\t20093\t\"Kearny County, KS\"\t20093\n\"Kearny County, KS\"\t20093\t\"Scott County, KS\"\t20171\n\"Kearny County, KS\"\t20093\t\"Stanton County, KS\"\t20187\n\"Kearny County, KS\"\t20093\t\"Wichita County, KS\"\t20203\n\"Kingman County, KS\"\t20095\t\"Barber County, KS\"\t20007\n\"Kingman County, KS\"\t20095\t\"Harper County, KS\"\t20077\n\"Kingman County, KS\"\t20095\t\"Kingman County, KS\"\t20095\n\"Kingman County, KS\"\t20095\t\"Pratt County, KS\"\t20151\n\"Kingman County, KS\"\t20095\t\"Reno County, KS\"\t20155\n\"Kingman County, KS\"\t20095\t\"Sedgwick County, KS\"\t20173\n\"Kingman County, KS\"\t20095\t\"Sumner County, KS\"\t20191\n\"Kiowa County, KS\"\t20097\t\"Barber County, KS\"\t20007\n\"Kiowa County, KS\"\t20097\t\"Clark County, KS\"\t20025\n\"Kiowa County, KS\"\t20097\t\"Comanche County, KS\"\t20033\n\"Kiowa County, KS\"\t20097\t\"Edwards County, KS\"\t20047\n\"Kiowa County, 
